vi "ethernet_ip.vi"(0 "EIP":T2, 1 "network path":string="192.168.1.10", 5 "Number of Elements":u32=1, 7 "Tag Name":string, 9 "data in":variant, 11 "error in (no error)":errorcluster, 12 "Session in":T1) -> (2 "8INT out":i8[](array[numeric]), 3 "16INT out":i16[](array[numeric]), 4 "32INT out":i32[](array[numeric]), 6 "SGL out":sgl[](array[numeric]), 8 "BOOL out":bool[](array[boolean]), 10 "STRING out":string, 13 "Session out":T1, 14 "RAW U8 out":u8[](array[numeric]), 15 "error out":errorcluster)   [LabVIEW 2020]
uses:
  EIP.ctl
  <vilib>/ethernetip/ethernetip.llb/ethernetip.ctl
  <userlib>/_OpenG.lib/string/string.llb/Trim Whitespace (String)__ogtk.vi
  <vilib>/ethernetip/ethernetip.llb/EthernetIP Tag Read SINT.vi
  <vilib>/ethernetip/ethernetip.llb/EthernetIP Tag Read INT.vi
  <vilib>/ethernetip/ethernetip.llb/EthernetIP Tag Read DINT.vi
  <vilib>/ethernetip/ethernetip.llb/EthernetIP Tag Read REAL.vi
  <vilib>/ethernetip/ethernetip.llb/EthernetIP Tag Read BOOL.vi
  <vilib>/ethernetip/ethernetip.llb/EthernetIP Tag Read STRING.vi
  <vilib>/ethernetip/ethernetip.llb/EthernetIP Tag Read Raw.vi
  <vilib>/ethernetip/ethernetip.llb/EthernetIP Tag Write SINT.vi
  <vilib>/ethernetip/ethernetip.llb/EthernetIP Tag Write INT.vi
  <vilib>/ethernetip/ethernetip.llb/EthernetIP Tag Write DINT.vi
  <vilib>/ethernetip/ethernetip.llb/EthernetIP Tag Write REAL.vi
  <vilib>/ethernetip/ethernetip.llb/EthernetIP Tag Write BOOL.vi
  <vilib>/ethernetip/ethernetip.llb/EthernetIP Tag Write STRING.vi
  <vilib>/ethernetip/ethernetip.llb/EthernetIP Tag Write Raw.vi
  <vilib>/ethernetip/ethernetip.lvlib
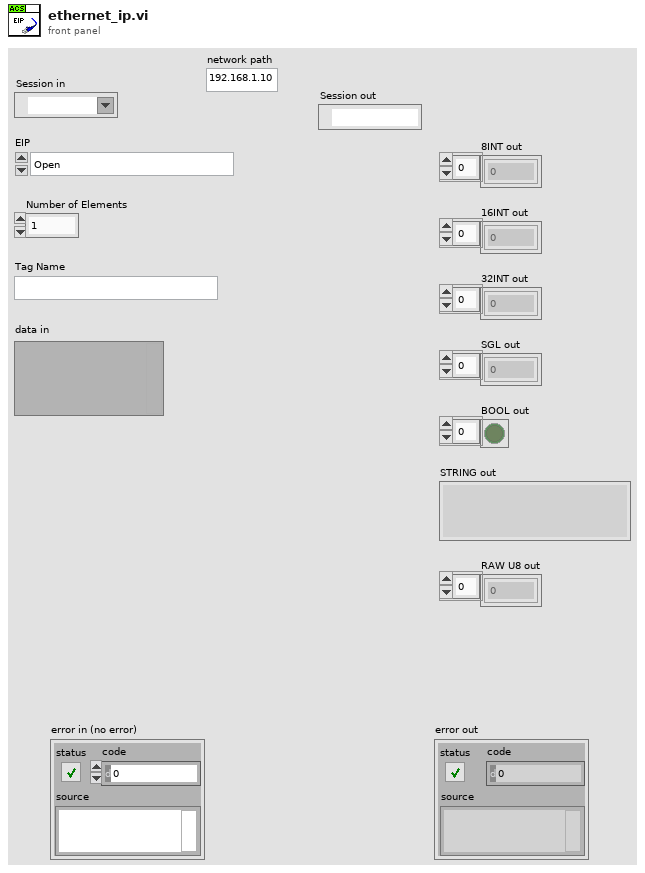
[diagram p1: front panel]
types:
  T1 = typedef "ethernetip.lvlib/ethernetip.ctl" = refnum<k21>
  T2 = typedef "EIP.ctl" = enum16{"Open", "Close", "Tag Read SINT", "Tag Read INT", "Tag Read DINT", "Tag Read REAL", "Tag Read BOOL", "Tag Read STRING", "Tag Read RAW", "Tag Write SINT", "Tag Write INT", "Tag Write DINT", "Tag Write REAL", "Tag Write BOOL", "Tag Write STRING", "Tag Write Raw"}
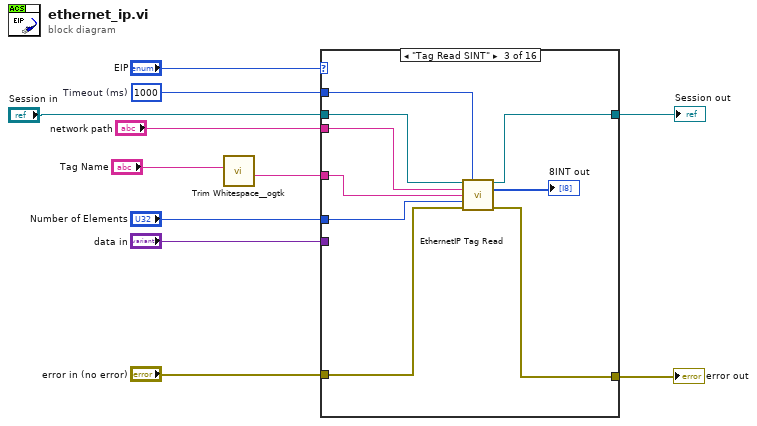
[diagram p0: block diagram]
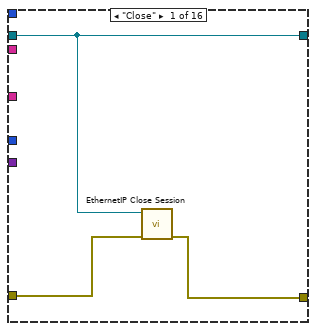
[diagram p2: hidden frame]
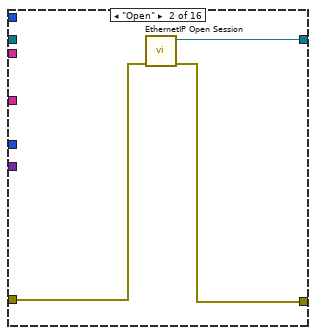
[diagram p3: hidden frame]
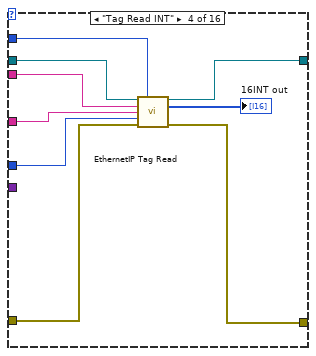
[diagram p4: hidden frame]
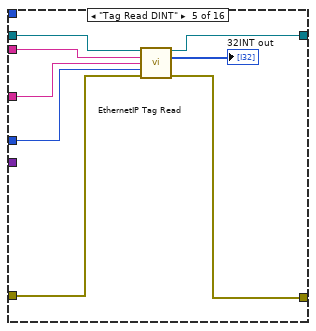
[diagram p5: hidden frame]
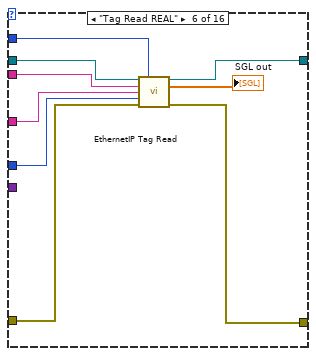
[diagram p6: hidden frame]
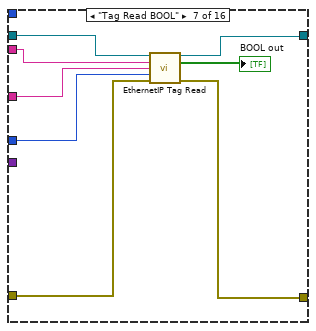
[diagram p7: hidden frame]
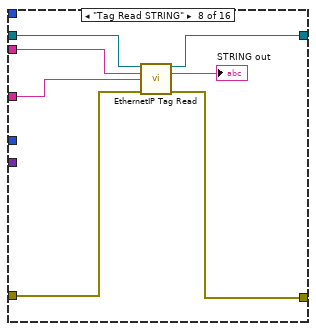
[diagram p8: hidden frame]
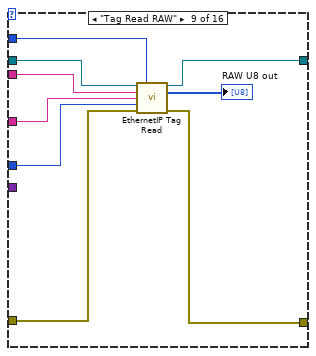
[diagram p9: hidden frame]
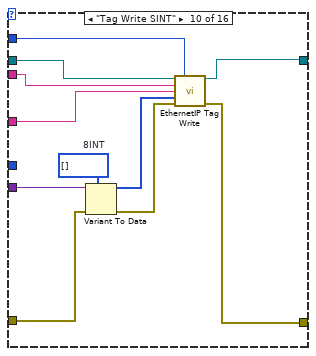
[diagram p10: hidden frame]
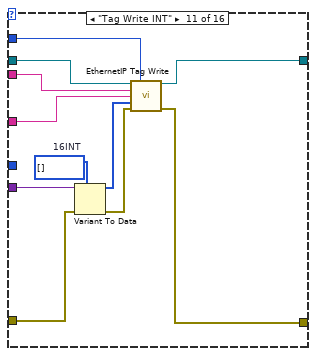
[diagram p11: hidden frame]
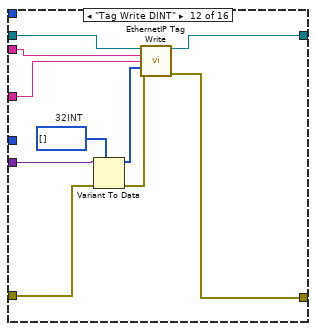
[diagram p12: hidden frame]
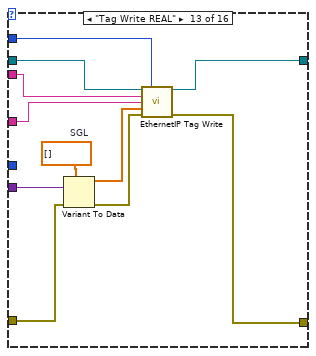
[diagram p13: hidden frame]
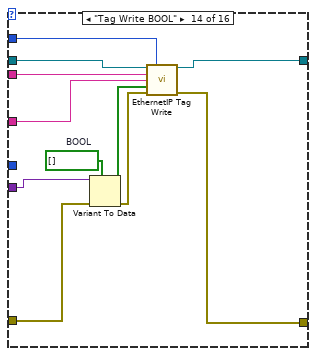
[diagram p14: hidden frame]
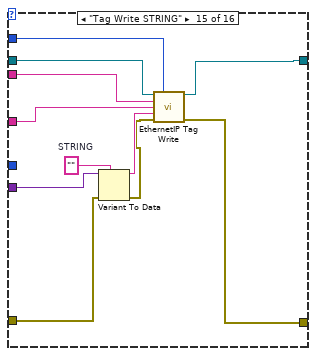
[diagram p15: hidden frame]
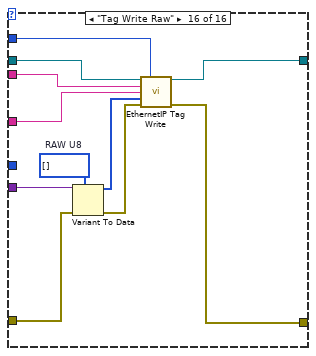
[diagram p16: hidden frame]
diagram:
  w6 = 1000  # Timeout (ms)
  n1 = call-poly <userlib>:"Trim Whitespace__ogtk.vi"("String in"="Tag Name") -> ("String out"=w1:string)  [unwired: 6 in]
  n2 = case shown="\"Tag Read SINT\"" "EIP" {
    tunnel: [w12 w17 w23 w34 w40 w48 w59 w66 w74 w86 w96 w107 w116 w128 w139 w150] -> w2
    tunnel: "Session in" -> [w12 _ w25 w35 w42 w52 w60 w67 w75 w87 w97 w108 w118 w130 w140 w151]
    tunnel: "Number of Elements" -> [_ _ w26 w30 w38 w49 w54 _ w69 _ _ _ _ _ _ _]
    tunnel: w1 -> [_ _ w24 w31 w39 w50 w55 w62 w70 w85 w95 w105 w117 w129 w138 w149]
    tunnel: "network path" -> [_ _ w22 w32 w41 w51 w56 w63 w71 w77 w88 w99 w109 w120 w131 w142]
    tunnel: "error in (no error)" -> [w14 w16 w21 w29 w37 w47 w58 w65 w73 w80 w90 w101 w111 w122 w133 w144]
    tunnel: [w13 w15 w20 w28 w36 w46 w57 w64 w72 w84 w94 w106 w115 w126 w137 w148] -> w7
    tunnel: w6 -> [_ _ w18 w27 _ w45 _ _ w76 w78 w98 _ w119 w127 w141 w152]
    tunnel: "data in" -> [_ _ _ _ _ _ _ _ _ w82 w92 w103 w114 w125 w136 w147]
    frame "Close" {
      n3 = call <vilib>:"EthernetIP Close Session.vi"("error in"=w14, "Session in"=w12) -> ("error out"=w13:errorcluster)  [unwired: 9 in]
    }
    frame "Open" {
      n4 = call <vilib>:"EthernetIP Open Session.vi"("error in"=w16) -> ("error out"=w15:errorcluster, "Session out"=w17:T1)  [unwired: 9 in]
    }
    frame "Tag Read SINT" {
      n5 = call-poly <vilib>:"EthernetIP Tag Read.vi"("Session in"=w25, "Timeout (ms)"=w18, "Network Path"=w22, "Tag Name"=w24, "Number of Elements"=w26, "error in"=w21) -> ("Session out"=w23:T1, "Data"=→"8INT out":i8[], "error out"=w20:errorcluster)  [unwired: 7 in]
    }
    frame "Tag Read INT" {
      n6 = call-poly <vilib>:"EthernetIP Tag Read.vi"("Session in"=w35, "Timeout (ms)"=w27, "Network Path"=w32, "Tag Name"=w31, "Number of Elements"=w30, "error in"=w29) -> ("Session out"=w34:T1, "Data"=→"16INT out":i16[], "error out"=w28:errorcluster)  [unwired: 7 in]
    }
    frame "Tag Read DINT" {
      n7 = call-poly <vilib>:"EthernetIP Tag Read.vi"("Session in"=w42, "Network Path"=w41, "Tag Name"=w39, "Number of Elements"=w38, "error in"=w37) -> ("Session out"=w40:T1, "Data"=→"32INT out":i32[], "error out"=w36:errorcluster)  [unwired: 8 in]
    }
    frame "Tag Read REAL" {
      n8 = call-poly <vilib>:"EthernetIP Tag Read.vi"("Session in"=w52, "Timeout (ms)"=w45, "Network Path"=w51, "Tag Name"=w50, "Number of Elements"=w49, "error in"=w47) -> ("Session out"=w48:T1, "Data"=→"SGL out":sgl[], "error out"=w46:errorcluster)  [unwired: 7 in]
    }
    frame "Tag Read BOOL" {
      n9 = call-poly <vilib>:"EthernetIP Tag Read.vi"("Session in"=w60, "Network Path"=w56, "Tag Name"=w55, "Number of Elements"=w54, "error in"=w58) -> ("Session out"=w59:T1, "Data"=→"BOOL out":bool[], "error out"=w57:errorcluster)  [unwired: 8 in]
    }
    frame "Tag Read STRING" {
      n10 = call-poly <vilib>:"EthernetIP Tag Read.vi"("Session in"=w67, "Network Path"=w63, "Tag Name"=w62, "error in"=w65) -> ("Session out"=w66:T1, "Data"=→"STRING out":string, "error out"=w64:errorcluster)  [unwired: 9 in]
    }
    frame "Tag Read RAW" {
      n11 = call-poly <vilib>:"EthernetIP Tag Read.vi"("Session in"=w75, "Timeout (ms)"=w76, "Network Path"=w71, "Tag Name"=w70, "Number of Elements"=w69, "error in"=w73) -> ("Session out"=w74:T1, "Data"=→"RAW U8 out":u8[], "error out"=w72:errorcluster)  [unwired: 7 in]
    }
    frame "Tag Write SINT" {
      w83 = i8[] []  # 8INT
      n12 = Variant To Data(error in=w80, type=w83, Variant=w82) -> (data=w81:i8[], error out=w79:errorcluster)
      n13 = call-poly <vilib>:"EthernetIP Tag Write.vi"("Session in"=w87, "Timeout (ms)"=w78, "Network Path"=w77, "Tag Name"=w85, "Data"=w81, "error in"=w79) -> ("Session out"=w86:T1, "error out"=w84:errorcluster)  [unwired: 8 in]
    }
    frame "Tag Write INT" {
      w93 = i16[] []  # 16INT
      n14 = Variant To Data(error in=w90, type=w93, Variant=w92) -> (data=w91:i16[], error out=w89:errorcluster)
      n15 = call-poly <vilib>:"EthernetIP Tag Write.vi"("Session in"=w97, "Timeout (ms)"=w98, "Network Path"=w88, "Tag Name"=w95, "Data"=w91, "error in"=w89) -> ("Session out"=w96:T1, "error out"=w94:errorcluster)  [unwired: 8 in]
    }
    frame "Tag Write DINT" {
      w104 = i32[] []  # 32INT
      n16 = Variant To Data(error in=w101, type=w104, Variant=w103) -> (data=w102:i32[], error out=w100:errorcluster)
      n17 = call-poly <vilib>:"EthernetIP Tag Write.vi"("Session in"=w108, "Network Path"=w99, "Tag Name"=w105, "Data"=w102, "error in"=w100) -> ("Session out"=w107:T1, "error out"=w106:errorcluster)  [unwired: 9 in]
    }
    frame "Tag Write REAL" {
      w113 = sgl[] []  # SGL
      n18 = Variant To Data(error in=w111, type=w113, Variant=w114) -> (data=w112:sgl[], error out=w110:errorcluster)
      n19 = call-poly <vilib>:"EthernetIP Tag Write.vi"("Session in"=w118, "Timeout (ms)"=w119, "Network Path"=w109, "Tag Name"=w117, "Data"=w112, "error in"=w110) -> ("Session out"=w116:T1, "error out"=w115:errorcluster)  [unwired: 8 in]
    }
    frame "Tag Write BOOL" {
      w124 = bool[] []  # BOOL
      n20 = Variant To Data(error in=w122, type=w124, Variant=w125) -> (data=w123:bool[], error out=w121:errorcluster)
      n21 = call-poly <vilib>:"EthernetIP Tag Write.vi"("Session in"=w130, "Timeout (ms)"=w127, "Network Path"=w120, "Tag Name"=w129, "Data"=w123, "error in"=w121) -> ("Session out"=w128:T1, "error out"=w126:errorcluster)  [unwired: 8 in]
    }
    frame "Tag Write STRING" {
      w135 = ""  # STRING
      n22 = Variant To Data(error in=w133, type=w135, Variant=w136) -> (data=w134:string, error out=w132:errorcluster)
      n23 = call-poly <vilib>:"EthernetIP Tag Write.vi"("Session in"=w140, "Timeout (ms)"=w141, "Network Path"=w131, "Tag Name"=w138, "Data"=w134, "error in"=w132) -> ("Session out"=w139:T1, "error out"=w137:errorcluster)  [unwired: 8 in]
    }
    frame "Tag Write Raw" {
      w146 = u8[] []  # RAW U8
      n24 = Variant To Data(error in=w144, type=w146, Variant=w147) -> (data=w145:u8[], error out=w143:errorcluster)
      n25 = call-poly <vilib>:"EthernetIP Tag Write.vi"("Session in"=w151, "Timeout (ms)"=w152, "Network Path"=w142, "Tag Name"=w149, "Data"=w145, "error in"=w143) -> ("Session out"=w150:T1, "error out"=w148:errorcluster)  [unwired: 8 in]
    }
  }
  "error out" <- w7
  "Session out" <- w2
